vi "TestGraph.vi"() -> ()   [LabVIEW 2016, in "M1M3SupportEUI_Views.lvlib"]
uses:
  M1M3SupportEUI_Views.lvlib
  <vilib>/Math Plots/3D Math Plots/3D Scatter/3D Scatter XCtrl/3D Scatter.xctl
  <vilib>/Utility/miscctls.llb/LVPoint32TypeDef.ctl
  <vilib>/Math Plots/3D Math Plots/3D Scatter/3D Scatter Datatype/Public/Plot Helper (Vector).vi
  <vilib>/Math Plots/3D Math Plots/3D Scatter/3D Scatter Datatype/3D Scatter Datatype.lvclass
panel:
  out "stop":bool
  out "Coords":T1
  out "X Position":sgl
  out "Y Position":sgl
  in  "stop":bool
  out "3D Scatter":refnum<class "3D Plot Datatype.lvclass">[](xcontrol)
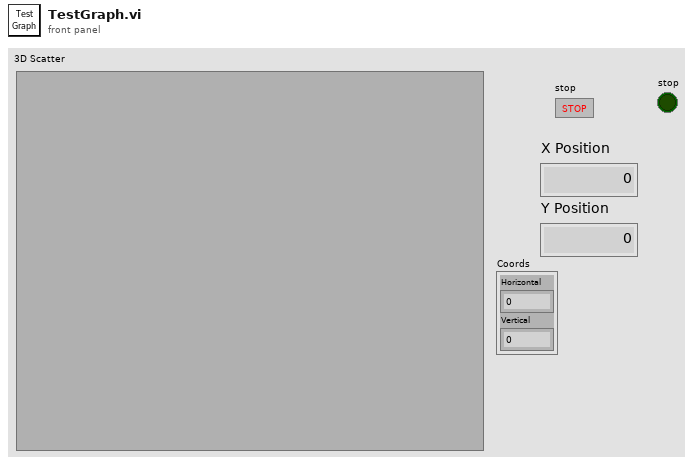
[diagram p1: front panel]
types:
  T1 = typedef "LVPoint32TypeDef.ctl" = cluster{"Horizontal":i32, "Vertical":i32}
  T2 = typedef "3D Plot.lvclass/Cursor Property Array.ctl" = T3[]
  T3 = typedef "3D Plot.lvclass/Cursor Property.ctl" = cluster{"Cursor Visible":bool, "Cursor Enable":bool, "Cursor Position":T4, "Cursor Point":T5, "Cursor Line":T7, "Cursor Plane":T9, "Cursor Text":T10}
  T4 = typedef "3D Plot.lvclass/Cursor Position.ctl" = cluster{"Cursor Plot ID":i32, "Cursor X":sgl, "Cursor Y":sgl, "Cursor Z":sgl, "Cursor Snap To":enum16{"Fixed", "Nearest Plot", "Snap to Plot"}}
  T5 = typedef "3D Plot.lvclass/Cursor Point.ctl" = cluster{"Cursor Point Color":u32, "Cursor Point Size":sgl, "Cursor Point Style":T6}
  T6 = typedef "3D Plot.lvclass/Sprite Type.ctl" = enum16{"None", "Empty Square", "Solid Square", "Empty Diamond", "Solid Diamond", "Empty Circle", "Solid Circle", "Asterisk", "Bold X", "Wireframe Sphere", "Solid Sphere", "Wireframe Cube", "Solid Cube"}
  T7 = typedef "3D Plot.lvclass/Cursor Line.ctl" = cluster{"Cursor Line Color":u32, "Cursor Line Width":sgl, "Cursor Line Style":T8}
  T8 = typedef "3D Plot.lvclass/Line Type.ctl" = enum16{"None", "Solid", "Dash", "Dot", "Dash Dot"}
  T9 = typedef "3D Plot.lvclass/Cursor Plane.ctl" = cluster{"Cursor Plane Color":u32, "Cursor Plane Opacity":sgl, "Draw Cursor Plane X-Z":bool, "Draw Cursor Plane Y-Z":bool, "Draw Cursor Plane X-Y":bool}
  T10 = typedef "3D Plot.lvclass/Cursor Text.ctl" = cluster{"Cursor Text":string, "Cursor Text Size":u16, "Cursor Show Position":bool, "Cursor Show Name":bool, "Cursor Text Color":u32, "Background Color":u32, "Background Opacity":sgl}
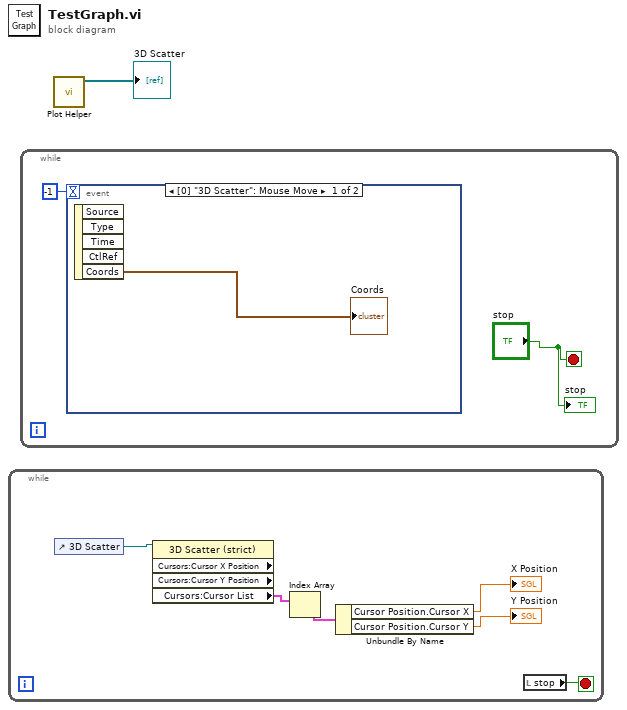
[diagram p0: block diagram]
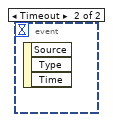
[diagram p2: hidden frame]
diagram:
  n1 = while {
    stop <- w7 stop-if-true
    n2 = control-ref of="3D Scatter"() -> (w2:refnum<vi>)
    n3 = property class="3D Scatter (strict)" props=["Cursors:Cursor X Position", "Cursors:Cursor Y Position", "Cursors:Cursor List"](reference=w2) -> ("Cursors:Cursor List"=w6:T2)  [unwired: 1 in, 4 out]
    n4 = Index Array(array=w6) -> (element=w5:T3)  [unwired: 1 in]
    n5 = Unbundle By Name(w5) -> ("Cursor Position.Cursor X"=→"X Position":sgl, "Cursor Position.Cursor Y"=→"Y Position":sgl)
    n6 = local read "stop"() -> (w7:bool)
  }
  n7 = while {
    stop <- "stop" stop-if-true
    n8 = event shown="[0] \"3D Scatter\": Mouse Move" {
      selector: _ -> [_ _]
      dyn-events: _ -> [_ _]
      timeout: -1 -> [_ _]
      event "3D Scatter": Mouse Move {
        n9 = event-data() -> ("Coords"=→"Coords":T1)  [unwired: 1 in, 4 out]
      }
      event Timeout {
        n10 = event-data() -> ()  [unwired: 1 in, 3 out]
      }
    }
    "stop" <- "stop"
  }
  n11 = call-poly <vilib>:"Plot Helper.vi"() -> ("3D Plot lvclass Array out"=→"3D Scatter":refnum<class "3D Plot Datatype.lvclass">[])  [unwired: 6 in, 5 out]
